vi "Arm_stage_var.vi"() -> ()   [LabVIEW 2019]
panel:
  in  "Arm stage":dbl
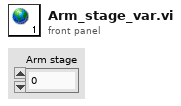
[diagram p1: front panel]
diagram:
